vi "Dashboard Main.vi"() -> ()   [LabVIEW 2013]
uses:
  <vilib>/Rock Robotics/WPI/Camera/WPI_CameraSettings Read MJPG.ctl
  <vilib>/Rock Robotics/WPI/Camera/WPI_CameraImageSize.ctl
panel:
  in  "Enable":bool
  in  "Tab Control":enum32{"In Match", "In Pit"}(tab)
  out "Number of shots taken":dbl
  out "Kinect Status":bool
  out "Ball In Intake?":bool
  out "Shooter is Front":bool
  out "Intake is Front":bool
  out "State Machine":bool
  out "Manual":bool
  out "Driver Can Controll":cluster{"X":bool, "Y":bool, "Rotate":bool}
  in  "Alliance":bool
  out "Red":bool
  in  "Reload":bool
  out "Error":bool
  out "Drive Mode":u16
  out "Auto Mode":u16
  out "Track X complete?":bool
  out "Track X":bool
  out "Anti-Rotate On?":bool
  out "Driver Controlled":bool
  out "Track X Error":dbl
  out "slow turn?":bool
  out "Kinect Players":i8
  out "Player":bool
  out "HighPressure":dbl format="%#_3g"
  out "Left encoder count":dbl
  out "Right encoder count":dbl
  out "Ball Voltage":dbl
  out "Cat Down Voltage":dbl
  out "SM state":string
  out "YawGyro":dbl
  out "Auto Distance":dbl
  out "RTAngle":dbl
  out "LTAngle":dbl
  out "StartFiringTime":dbl
  out "RotatePWR":dbl
  out "StrafePWR":dbl
  out "FireDelay":dbl
  out "TussShot":dbl
  out "Image 2":T1(plugin-control)
  in  "Tabbed Info":T2(tab)
  in  "Std Devs 2":cluster{"Hue":dbl, "Sat":dbl, "Val":dbl}={"Hue"=4.0, "Sat"=6.0, "Val"=4.0}
  in  "Targets":i32=3
  in  "Area Size Limit % 2":dbl=0.4 format="%#_13g"
  in  "Score Cutoff 2":dbl(slide)=70.58823529411765 scale=0.0..100.0
  out "Bandwidth (Mbps) 2":dbl
  in  "Camera Settings 2":T3={"fps"=15, "compression"=30, "Image Size"=enum."160x120"}
  in  "Camera IP 2":string="10.8.36.11"
  in  "Color Components 2":T5={"Hue"={243.23333311080933, 20.233333110809326}, "Sat"={125.60287475585938, 242.93045043945312}, "Val"={83.88507843017578, 225.38158416748047}} {"Val" scale=0.0..255.0; "Sat" scale=0.0..255.0; "Hue" scale=0.0..255.0 scale format="%#_3g"}
  out "Fitted Mask":T1(plugin-control)
  out "Initial Mask":T1(plugin-control)
  in  "Annotations":enum16{"None", "Good", "All"}(ring)=enum."Good"
  out "Ranked Objects":T6(array[cluster]) {"Score" format="%#.1g"}
  in  "Line 3":i32(knob) scale=-160.0..160.0
  in  "Line 4":i32(knob)=96 scale=0.0..160.0
  in  "Write Ball Red":bool
  in  "Write Ball Blue":bool
  # "Red"
  # "Blue"
  # "Ranking Colors:\n1. green\n2. cyan\n3. magenta\n4. orange"
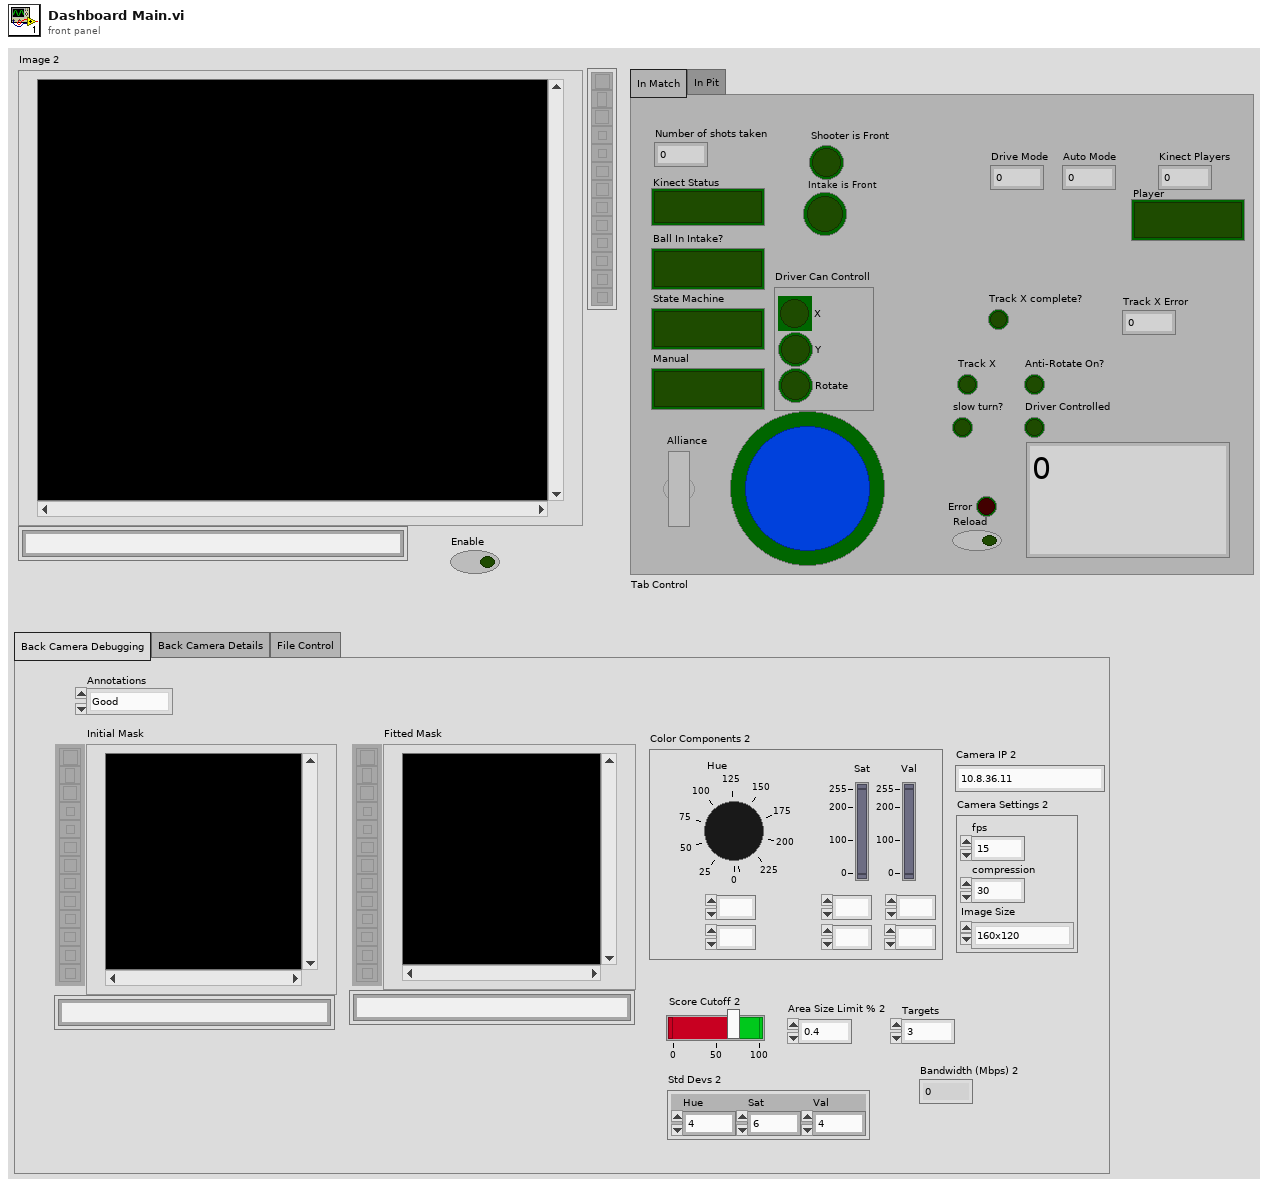
[diagram p1: front panel]
types:
  T1 = typedef "IMAQ Image.ctl" = refnum<image>
  T2 = enum32{"Back Camera Debugging", "Back Camera Details", "File Control"}
  T3 = typedef "WPI_CameraSettings Read MJPG.ctl" = cluster{"fps":i32, "compression":i32, "Image Size":T4}
  T4 = typedef "WPI_CameraImageSize.ctl" = enum16{"640x480", "320x240", "160x120"}
  T5 = cluster{"Hue":cluster{dbl, dbl}, "Sat":cluster{dbl, dbl}, "Val":cluster{dbl, dbl}}
  T6 = cluster{"Score":sgl, "Fitted Circle":cluster{"Center":cluster{"X":sgl, "Y":sgl}, "Radius":dbl, "Circle Rect":cluster{"L":sgl, "T":sgl, "R":sgl, "B":sgl}, "Roundness":dbl, "SNR (dB)":dbl}, "Search Rect":cluster{"L":sgl, "T":sgl, "R":sgl, "B":sgl}, "Details":cluster{"Edge":sgl, "Area":sgl, "Circ":sgl, "Diam":sgl}}[]
  T7 = cluster{cluster{"HueMin":i32, "HueMax":i32}, cluster{"SatMin":i32, "SatMax":i32}, cluster{"LumMin":i32, "LumMax":i32}}
  T8 = typedef "Image Type" = u32
  T9 = cluster{cluster{i32, i32}, cluster{"Line 4":i32, i32}}
  T10 = cluster{"Circle Found":bool, "Fitted Circle":cluster{"Center":cluster{"X":sgl, "Y":sgl}, "Radius":dbl, "Center":cluster{"X":sgl, "Y":sgl}, "Radius":dbl, "Roundness":dbl, "Strength":dbl, "SNR (dB)":dbl}, "Array":dbl[], "Sorted Data":dbl[][]}[]
  T11 = cluster{cluster{dbl, dbl}, cluster{dbl, dbl}, cluster{dbl, dbl}}
  T12 = cluster{"Score":dbl, "Fitted Circle":cluster{"Center (Pixels)":cluster{"X":sgl, "Y":sgl}, "Radius (Pixels)":dbl, "Circle Rect":cluster{"Left":sgl, "Top":sgl, "Right":sgl, "Bottom":sgl}, "Roundness (RW)":dbl, "Average SNR (dB)":dbl}, "Search Rect":cluster{"Left":sgl, "Top":sgl, "Right":sgl, "Bottom":sgl}, "Details":cluster{"Edges":sgl, "Circ/Rect":sgl, "Diam/Diam":sgl, "Circularity":sgl}}[]
  T13 = cluster{"Score":dbl, "Fitted Circle":cluster{"Center (Pixels)":cluster{"X":sgl, "Y":sgl}, "Radius (Pixels)":dbl, "Circle Rect":cluster{"Left":sgl, "Top":sgl, "Right":sgl, "Bottom":sgl}, "Roundness (RW)":dbl, "Average SNR (dB)":dbl}, "Search Rect":cluster{"Left":sgl, "Top":sgl, "Right":sgl, "Bottom":sgl}, "Details":cluster{"Edges":sgl, "Circ/Rect":sgl, "Diam/Diam":sgl, "Circularity":sgl}}
  T14 = cluster{"Center (Pixels)":cluster{"X":sgl, "Y":sgl}, "Radius (Pixels)":dbl, "Circle Rect":cluster{"Left":sgl, "Top":sgl, "Right":sgl, "Bottom":sgl}, "Roundness (RW)":dbl, "Average SNR (dB)":dbl}
  T15 = cluster{"driverButton10":bool, "State Machine State":u16, "Ball Voltage":dbl, "Ball Voltage":dbl, "driverButton10":bool, "State Machine State":u16, "Ball Voltage":dbl, "State Machine State":u16, "driverButton10":bool, "Ball Voltage":dbl, "Ball Voltage":dbl, "Ball Voltage":dbl, "driverButton10":bool, "driverButton10":bool, "driverButton10":bool, "driverButton10":bool, "Ball Voltage":dbl, "Ball Voltage":dbl, "Ball Voltage":dbl, "Ball Voltage":dbl, "Ball Voltage":dbl, "Ball Voltage":dbl, "Ball Voltage":dbl, "Ball Voltage":dbl, "Ball Voltage":dbl}
  T16 = cluster{i8, "driverButton10":bool, "Ball Voltage":dbl}
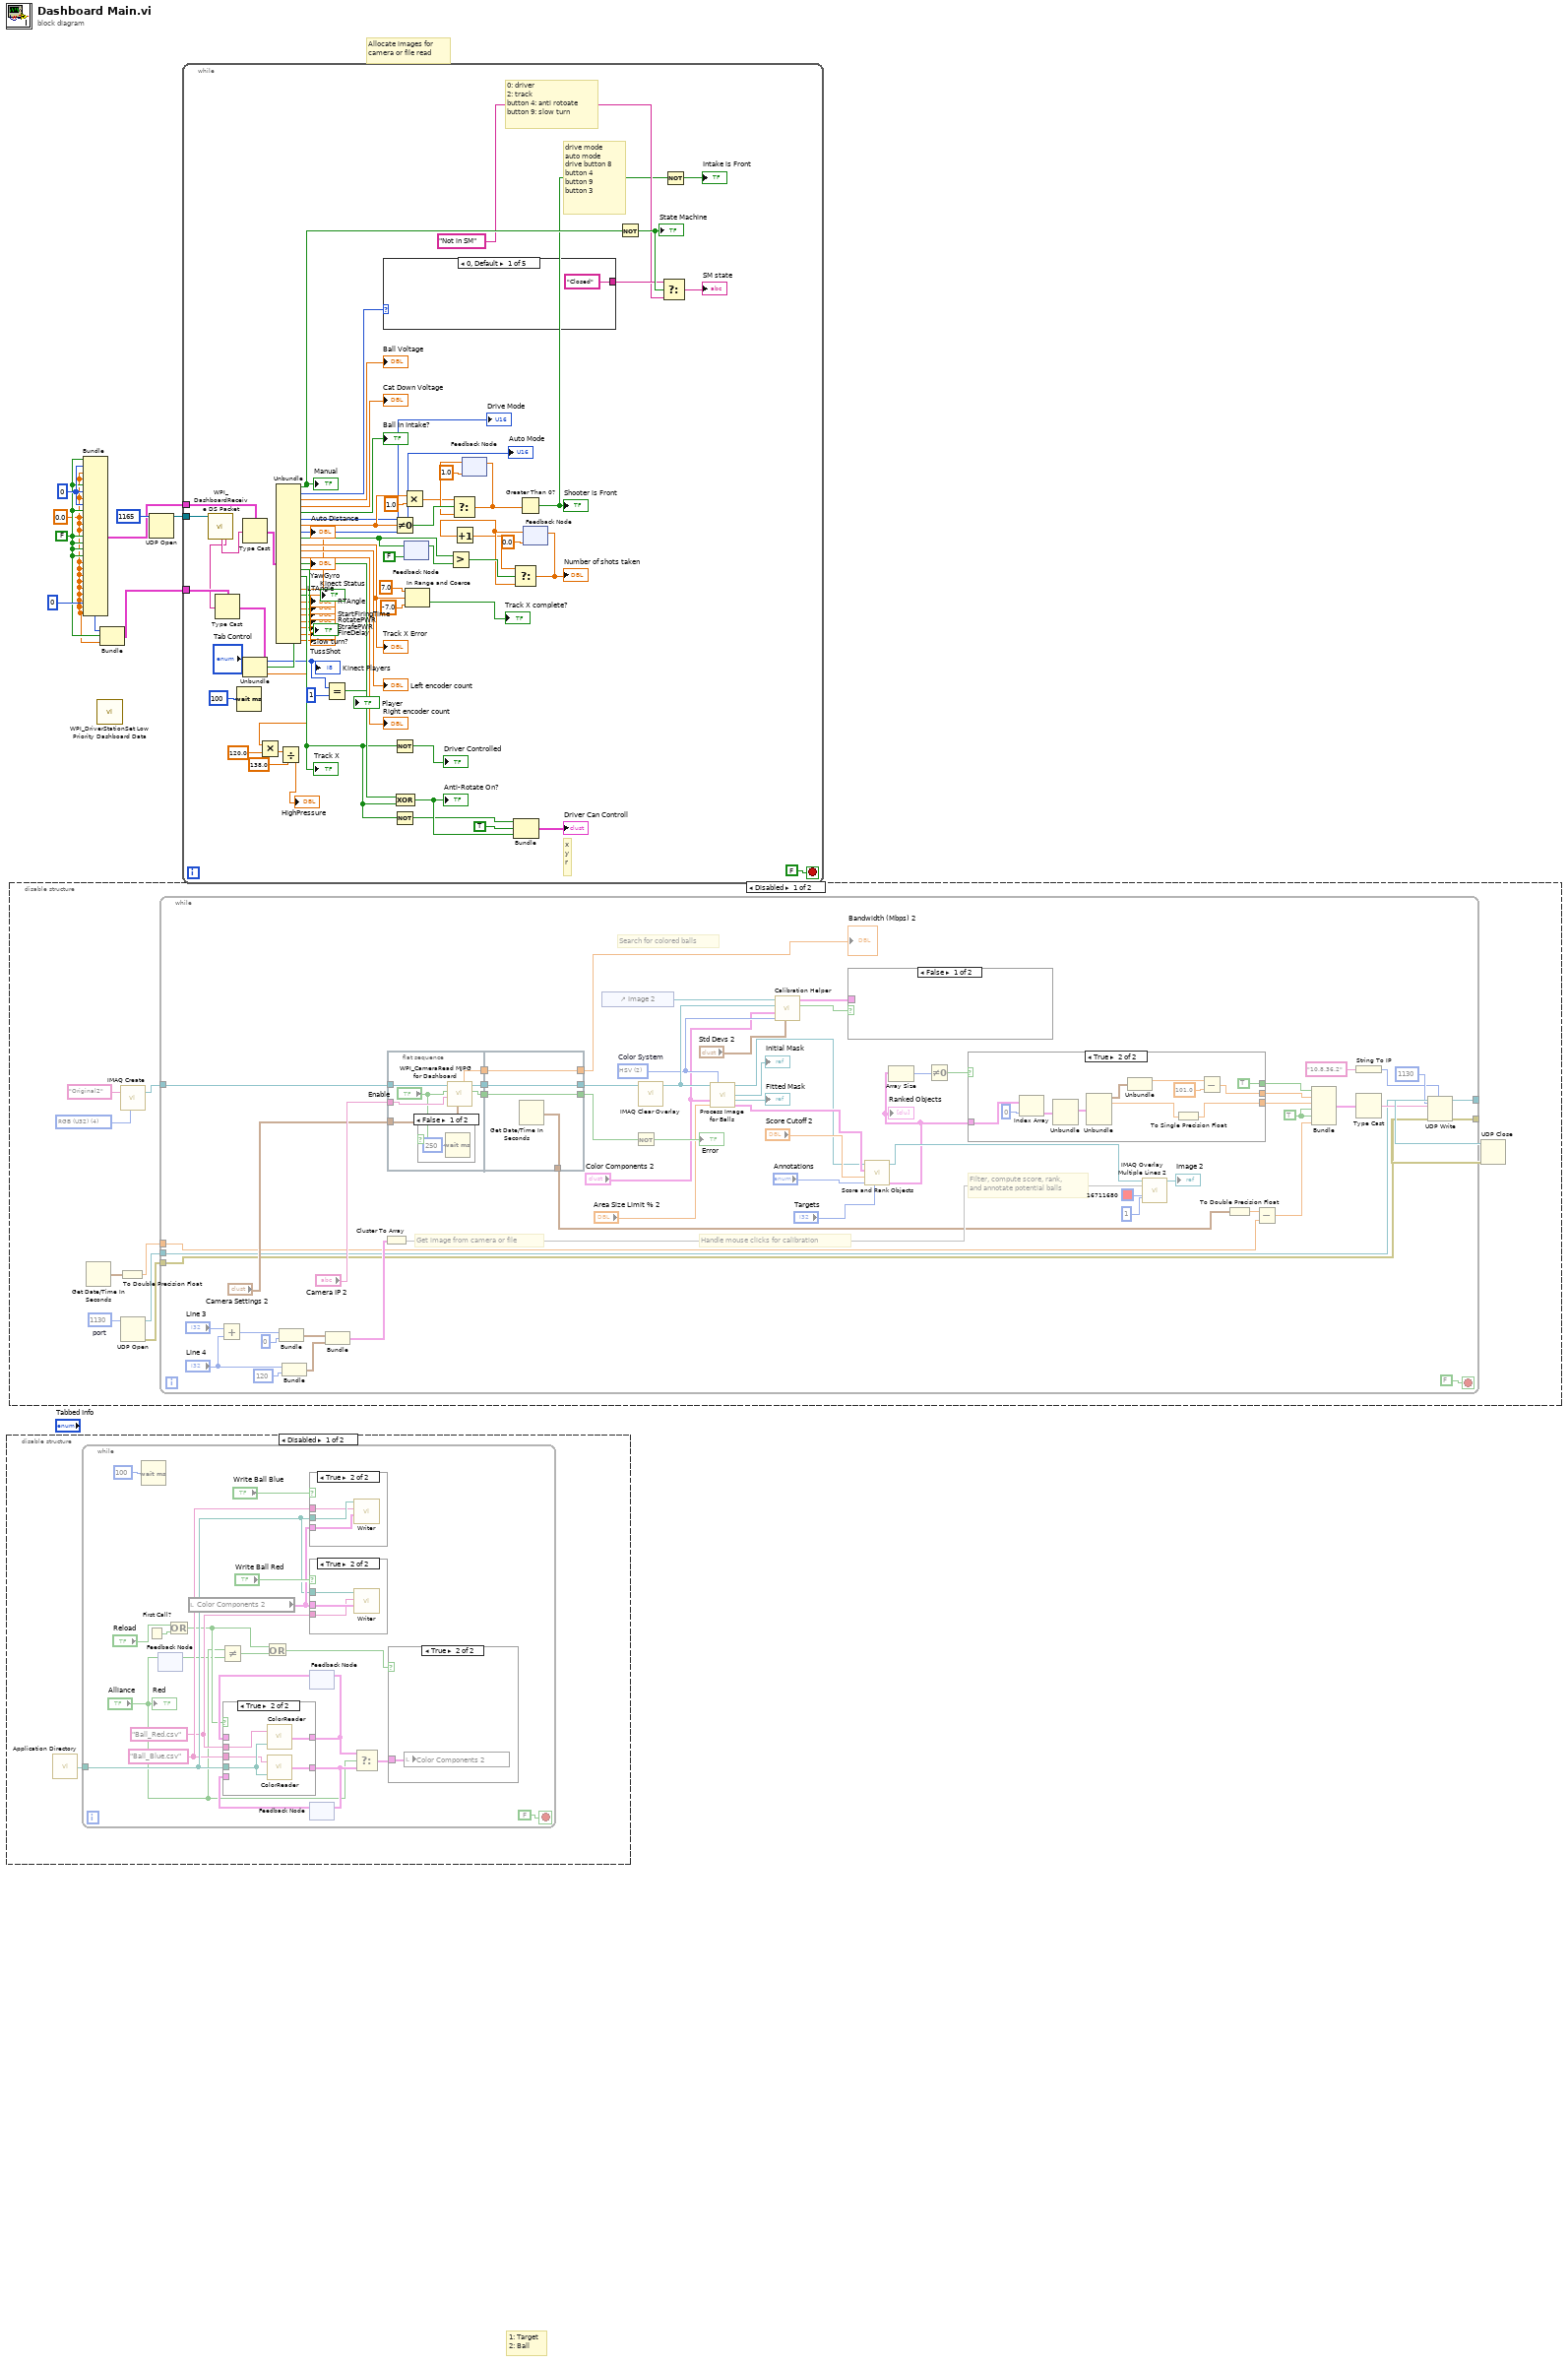
[diagram p0: block diagram]
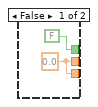
[diagram p8: hidden frame]
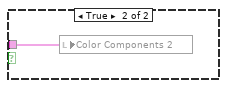
[diagram p9: hidden frame]
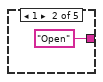
[diagram p11: hidden frame]
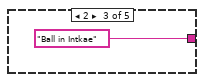
[diagram p12: hidden frame]
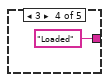
[diagram p13: hidden frame]
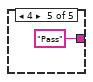
[diagram p14: hidden frame]
diagram:
  w3 = FALSE ("driverButton10")
  w1 = 0.0 ("Ball Voltage")
  w8 = u16 0 ("State Machine State")
  # "1: Target\n2: Ball"
  # "Allocate images for\ncamera or file read"
  n1 = disable-structure shown="Disabled" {
    frame Disabled {
      n2 = call <vilib>:"Application Directory.vi"() -> ("Application Directory"=w9:path)
      n3 = while {
        tunnel: w9 -> [w25]
        stop <- FALSE stop-if-true
        w21 = "Ball_Red.csv" ("FileName")
        w22 = "Ball_Blue.csv" ("FileName")
        n4 = Wait (ms)(milliseconds to wait=u32 100) -> ()  [unwired: 1 out]
        n5 = First Call?() -> (First Call?: T/F=w24:bool)
        n6 = feedback-in #1("Alliance") -> ()
        n7 = feedback #1() -> (w11:bool)  [unwired: 1 in]
        n8 = Or(x="Reload", y=w24) -> (x .or. y?=w14:bool)
        n9 = local read "Color Components 2"() -> (w26:T5)
        n10 = Not Equal?(x="Alliance", y=w11) -> (x != y?=w13:bool)
        n11 = Or(x=w14, y=w13) -> (x .or. y?=w15:bool)
        n12 = case shown="True" "Write Ball Blue" {
          tunnel: w25 -> [_ w43]
          tunnel: w26 -> [_ w41]
          tunnel: w22 -> [_ w42]
          frame False {
          }
          frame True {
            n13 = call "Writer.vi"("output cluster"=w41, "FileName"=w42, "FilePath"=w43) -> ()  [unwired: 9 in]
          }
        }
        n14 = case shown="True" "Write Ball Red" {
          tunnel: w25 -> [_ w39]
          tunnel: w26 -> [_ w40]
          tunnel: w21 -> [_ w38]
          frame False {
          }
          frame True {
            n15 = call "Writer.vi"("output cluster"=w40, "FileName"=w38, "FilePath"=w39) -> ()  [unwired: 9 in]
          }
        }
        n16 = feedback #2() -> (w19:T7)  [unwired: 1 in]
        n17 = feedback #3() -> (w17:T7)  [unwired: 1 in]
        n18 = case shown="True" w14 {
          tunnel: w25 -> [_ w37]
          tunnel: w22 -> [_ w36]
          tunnel: w21 -> [_ w35]
          tunnel: [w32 w34] -> w20
          tunnel: [w31 w33] -> w18
          tunnel: w19 -> [w32 _]
          tunnel: w17 -> [w31 _]
          frame False {
          }
          frame True {
            n19 = call "ColorReader.vi"("file path (dialog if empty)"=w37, "name or relative path"=w35) -> ("output cluster"=w34:T7)
            n20 = call "ColorReader.vi"("file path (dialog if empty)"=w37, "name or relative path"=w36) -> ("output cluster"=w33:T7)
          }
        }
        n21 = feedback-in #2(w20) -> ()
        n22 = feedback-in #3(w18) -> ()
        n23 = Select(t=w20, s="Alliance", f=w18) -> (s? t:f=w16:T7)
        n24 = case shown="True" w15 {
          tunnel: w16 -> [_ w30]
          frame False {
          }
          frame True {
            n25 = local write "Color Components 2"(w30) -> ()
          }
        }
        "Red" <- "Alliance"
      }
    }
    frame Enabled {
    }
  }
  n26 = disable-structure shown="Disabled" {
    frame Disabled {
      w50 = u16 1130  # port
      w53 = T8 4 items=["Grayscale (U8)", "Grayscale (I16)", "Grayscale (SGL)", "Complex (CSG)", "RGB (U32)", "HSL (U32)", "RGB (U64)", "Grayscale (U16)"] ("Image Type")
      n27 = Get Date/Time In Seconds() -> (seconds since 1Jan1904=w49:timestamp)
      n28 = To Double Precision Float(number=w49) -> (double precision float=w48:dbl)
      n29 = call "IMAQ Create"("Image Name"="Original2", "Image Type"=w53) -> ("New Image"=w51:T1)  [unwired: 3 in, 1 out]
      n30 = UDP Open(11:w50) -> (port=w46:refnum<k16>, 0:w47:errorcluster)  [unwired: 4 in, 1 out]
      n31 = while {
        tunnel: w51 -> [w110]
        tunnel: w48 -> [w81]
        tunnel: w47 -> [w70]
        tunnel: w46 -> [w69]
        tunnel: [w68] -> w45
        tunnel: [w67] -> w44
        stop <- FALSE stop-if-true
        w79 = TRUE
        w104 = u16 2 items=["RGB", "HSL", "HSV", "HSI"]  # Color System
        # "Handle mouse clicks for calibration"
        # "Search for colored balls"
        # "Filter, compute score, rank,\nand annotate potential balls"
        # "Get image from camera or file"
        n32 = Add(x="Line 3", y="Line 4") -> (x+y=w83:i32)
        n33 = Bundle(w83, 0) -> (w94:cluster{i32, i32})  [unwired: 1 in]
        n34 = Bundle("Line 4"="Line 4", 120) -> (w93:cluster{"Line 4":i32, i32})  [unwired: 1 in]
        n35 = Bundle(w94, w93) -> (w86:T9)  [unwired: 1 in]
        n36 = Cluster To Array(cluster=w86) -> (array=w92:cluster{"Line 4":i32, i32}[])
        n37 = flat-sequence {
          tunnel: [w119] -> w64
          tunnel: w110 -> [w118]
          tunnel: "Camera IP 2" -> [w117]
          tunnel: [w116] -> w63
          tunnel: "Camera Settings 2" -> [w115]
          tunnel: [w114] -> w62
          tunnel: [w124] -> w112
          tunnel: w64 -> [w124]
          tunnel: [w123] -> w97
          tunnel: w63 -> [w123]
          tunnel: [w122] -> w95
          tunnel: w62 -> [w122]
          tunnel: [w121] -> w61
          frame #0 {
            n38 = case shown="False" "Enable" {
              frame False {
                n39 = Wait (ms)(milliseconds to wait=u32 250) -> ()  [unwired: 1 out]
              }
              frame True {
              }
            }
            n40 = call <vilib>:"WPI_CameraRead MJPG for Dashboard.vi"("Camera Settings"=w115, "Camera IP"=w117, "Enable"="Enable", "Refnum in"=w118) -> ("Active"=w116:bool, "Refnum out"=w119:T1, "Bandwidth (Mbps)"=w114:dbl)  [unwired: 4 in, 1 out]
          }
          frame #1 {
            n41 = Get Date/Time In Seconds() -> (seconds since 1Jan1904=w121:timestamp)
          }
        }
        n42 = control-ref of="Image 2"() -> (w103:refnum<vi>)
        n43 = Not(x=w97) -> (.not. x?=→"Error":bool)
        n44 = call "IMAQ Clear Overlay"("Image"=w112) -> ("Image Out"=w108:T1)  [unwired: 9 in, 1 out]
        n45 = call "Process Image for Balls.vi"("Src Image"=w108, "Color Mode 2"=w104, "Color"="Color Components 2", "Area Cutoff %"="Area Size Limit % 2") -> ("Src Image Out"=w56:T1, "First Threshold"=→"Initial Mask":T1, "Fitted"=→"Fitted Mask":T1, "Potential"=w57:T10)  [unwired: 8 in]
        n46 = call "Calibration Helper.vi"("Std Devs"="Std Devs 2", "Color Mode"=w104, "Color Components"="Color Components 2", "Image"=w108, "Image Ctl Refnum"=w103) -> ("Changed"=w100:bool, "output color"=w102:T11)  [unwired: 5 in]
        n47 = case shown="False" w100 {
          tunnel: w102 -> [_ w138]
          frame False {
          }
          frame True {
            n48 = local write "Color Components 2"(w138) -> ()
          }
        }
        n49 = call "Score and Rank Objects.vi"("Targets"="Targets", "Annotations"="Annotations", "Score Limit"="Score Cutoff 2", "Object Info"=w57, "Image in"=w56) -> ("Object Info"=w54:T12, "Annotated Image"=w55:T1)  [unwired: 5 in]
        "Ranked Objects" <- w54
        n50 = Array Size(array=w54) -> (size(s)=w77:i32)
        n51 = Not Equal To 0?(x=w77) -> (x != 0?=w78:bool)
        n52 = case shown="True" w78 {
          tunnel: w54 -> [_ w136]
          tunnel: [FALSE TRUE] -> w74
          tunnel: [w125 w129] -> w75
          tunnel: [w125 w127] -> w76
          frame False {
            w125 = sgl 0.0
          }
          frame True {
            n53 = Index Array(array=w136, index=0) -> (element=w135:T13)
            n54 = Unbundle(w135) -> ("Fitted Circle"=w133:T14)  [unwired: 3 out]
            n55 = Unbundle(w133) -> ("Center (Pixels)"=w132:cluster{"X":sgl, "Y":sgl}, "Radius (Pixels)"=w128:dbl)  [unwired: 3 out]
            n56 = Unbundle(w132) -> ("X"=w131:sgl)  [unwired: 1 out]
            n57 = To Single Precision Float(number=w128) -> (single precision float=w127:sgl)
            n58 = Subtract(x=w131, y=sgl 101.0) -> (x-y=w129:sgl)
          }
        }
        n59 = call "IMAQ Overlay Multiple Lines 2"("Image"=w55, "Line End Points"=w92, "Color"=u32 16711680, "Width"=u32 1) -> ("Image Out"=→"Image 2":T1)  [unwired: 10 in, 1 out]
        n60 = To Double Precision Float(number=w61) -> (double precision float=w82:dbl)
        n61 = Subtract(x=w82, y=w81) -> (x-y=w80:dbl)
        n62 = Bundle(w74, w75, w76, w79, w79, w80) -> (w71:cluster{bool, sgl, sgl, bool, bool, dbl})  [unwired: 1 in]
        n63 = String To IP(1:"10.8.36.2" ("name")) -> (0:w65:u32)
        n64 = Type Cast(x=w71) -> (*(type *) &x=w72:string)  [unwired: 1 in]
        n65 = UDP Write(address=w65, port or service name=u16 1130, connection ID=w69, data in=w72, 8:w70) -> (error out=w67:errorcluster, 3:w68:refnum<k16>)  [unwired: 1 in]
        "Bandwidth (Mbps) 2" <- w95
      }
      n66 = UDP Close(connection ID=w45, 8:w44) -> ()  [unwired: 2 out]
    }
    frame Enabled {
    }
  }
  n67 = Bundle("driverButton10"=w3, "State Machine State"=w8, "Ball Voltage"=w1, "Ball Voltage"=w1, "driverButton10"=w3, "State Machine State"=w8, "Ball Voltage"=w1, "State Machine State"=w8, "driverButton10"=w3, "Ball Voltage"=w1, "Ball Voltage"=w1, "Ball Voltage"=w1, "driverButton10"=w3, "driverButton10"=w3, "driverButton10"=w3, "driverButton10"=w3, "Ball Voltage"=w1, "Ball Voltage"=w1, "Ball Voltage"=w1, "Ball Voltage"=w1, "Ball Voltage"=w1, "Ball Voltage"=w1, "Ball Voltage"=w1, "Ball Voltage"=w1, "Ball Voltage"=w1) -> (w5:T15)  [unwired: 1 in]
  n68 = call <vilib>:"WPI_DriverStationSet Low Priority Dashboard Data.vi"() -> ()  [unwired: 11 in, 1 out]
  n69 = Bundle(i8 0, "driverButton10"=w3, "Ball Voltage"=w1) -> (w2:T16)  [unwired: 1 in]
  n70 = UDP Open(11:u16 1165 ("port")) -> (port=w6:refnum<k16>)  [unwired: 4 in, 2 out]
  n71 = while {
    tunnel: w6 -> [w207]
    tunnel: w5 -> [w205]
    tunnel: w2 -> [w159]
    stop <- FALSE stop-if-true
    # "0: driver\n2: track\nbutton 4: anti rotoate\nbutton 9: slow turn"
    # "x\ny\nr"
    # "drive mode\nauto mode\ndrive button 8\nbutton 4\nbutton 9\nbutton 3"
    n72 = call <vilib>:"WPI_DashboardReceive DS Packet.vi"("Recv Socket"=w207) -> ("Low Priority User Data"=w206:string, "High Priority User Data"=w158:string)  [unwired: 1 in, 12 out]
    n73 = Type Cast(type=w159, x=w158) -> (*(type *) &x=w157:T16)
    n74 = Wait (ms)(milliseconds to wait=u32 100) -> ()  [unwired: 1 out]
    n75 = Type Cast(type=w205, x=w206) -> (*(type *) &x=w204:T15)
    n76 = Unbundle(w157) -> (w155:i8, "driverButton10"=→"Kinect Status":bool, "Ball Voltage"=w143:dbl)
    "Kinect Players" <- w155
    n77 = Multiply(x=w143, y=120.0) -> (x*y=w141:dbl)
    n78 = Unbundle(w204) -> ("driverButton10"=w203:bool, "State Machine State"=w202:u16, "Ball Voltage"=→"Ball Voltage":dbl, "Ball Voltage"=→"Cat Down Voltage":dbl, "driverButton10"=→"Ball In Intake?":bool, "State Machine State"=→"Drive Mode":u16, "Ball Voltage"=w186:dbl, "State Machine State"=→"Auto Mode":u16, "driverButton10"=w175:bool, "Ball Voltage"=w184:dbl, "Ball Voltage"=→"Left encoder count":dbl, "Ball Voltage"=→"Right encoder count":dbl, "driverButton10"=w167:bool, "driverButton10"=→"slow turn?":bool, "driverButton10"=w164:bool, "Ball Voltage"=→"YawGyro":dbl, "Ball Voltage"=→"Auto Distance":dbl, "Ball Voltage"=→"RTAngle":dbl, "Ball Voltage"=→"LTAngle":dbl, "Ball Voltage"=→"StartFiringTime":dbl, "Ball Voltage"=→"RotatePWR":dbl, "Ball Voltage"=→"StrafePWR":dbl, "Ball Voltage"=→"FireDelay":dbl, "Ball Voltage"=→"TussShot":dbl)  [unwired: 1 out]
    "Manual" <- w203
    "Track X" <- w164
    "Track X Error" <- w184
    n79 = Divide(x=w141, y=138.0) -> (x/y=→"HighPressure":dbl)
    n80 = Equal?(x=w155, y=i8 1) -> (x = y?=→"Player":bool)
    n81 = case shown="0, Default" w202 {
      tunnel: ["Closed" "Open" "Ball in Intkae" "Loaded" "Pass"] -> w200
      frame 0, Default {
      }
      frame 1 {
      }
      frame 2 {
      }
      frame 3 {
      }
      frame 4 {
      }
    }
    n82 = Not Equal To 0?(x=w186) -> (x != 0?=w194:bool)
    n83 = Not(x=w164) -> (.not. x?=→"Driver Controlled":bool)
    n84 = Not(x=w164) -> (.not. x?=w163:bool)
    n85 = Exclusive Or(1:w164, 2:w167) -> (0:w166:bool)
    "Anti-Rotate On?" <- w166
    n86 = Multiply(x=w186, y=1.0) -> (x*y=w190:dbl)
    n87 = feedback-in #4(w175) -> ()
    n88 = feedback #4(FALSE ("driverButton10")) -> (w174:bool)
    n89 = In Range and Coerce(upper limit=7.0, x=w184, lower limit=-7.0) -> (In Range?=→"Track X complete?":bool)  [unwired: 1 out]
    n90 = Greater?(x=w175, y=w174) -> (0:w172:bool)
    n91 = feedback #5(1.0) -> (w193:dbl)
    n92 = Select(t=w190, s=w194, f=w193) -> (s? t:f=w189:dbl)
    n93 = feedback-in #5(w189) -> ()
    n94 = Bundle(w163, TRUE, w166) -> (→"Driver Can Controll":cluster{bool, bool, bool})  [unwired: 1 in]
    n95 = Greater Than 0?(x=w189) -> (x > 0?=w187:bool)
    "Shooter is Front" <- w187
    n96 = feedback #6(0.0) -> (w171:dbl)
    n97 = Increment(x=w171) -> (x+1=w170:dbl)
    n98 = Select(t=w170, s=w172, f=w171) -> (s? t:f=w177:dbl)
    "Number of shots taken" <- w177
    n99 = feedback-in #6(w177) -> ()
    n100 = Not(x=w203) -> (.not. x?=w201:bool)
    "State Machine" <- w201
    n101 = Select(t=w200, s=w201, f="Not in SM") -> (s? t:f=→"SM state":string)
    n102 = Not(x=w187) -> (.not. x?=→"Intake is Front":bool)
  }
